vi "Read Controller Info.vi"(7 "Unit ID (A)":string="A", 8 "error in":errorcluster, 10 "Software Version":u8, 11 "VISA Session In":refnum<visa-resource-name>="Alicat") -> (0 "error out":errorcluster, 1 "Disabled Items\n(used with\"DisabledItems[]\" in the\nController Select property node)":i32[](array[numeric]), 2 "Controller Info out":T1={"Controller Full Scale"=nan, "Controller Select"=0, "Control Range"=enum."Normal"} {"Controller Select" items=["No controller"=0, "Volumetric Flow"=36, "Mass Flow"=37, "Absolute Pressure"=34, "Gauge Pressure"=38, "Differential Pressure"=39]}, 3 "VISA Session Out":refnum<visa-resource-name>)   [LabVIEW 2019]
doc: "Reads multiple registers to determine the Alicat controller settings required to run the \"Write Setpoint\" VI. Outputs the currently selected control variable, its full scale, and whether the full scale is inverted, normal, or bi-directional."
uses:
  <vilib>/Instr/_visa.llb/VISA Flush IO Buffer Mask.ctl
panel:
  # "SW Version defaults to 0. \nIf un-wired, it will call a \nsub-VI to check."
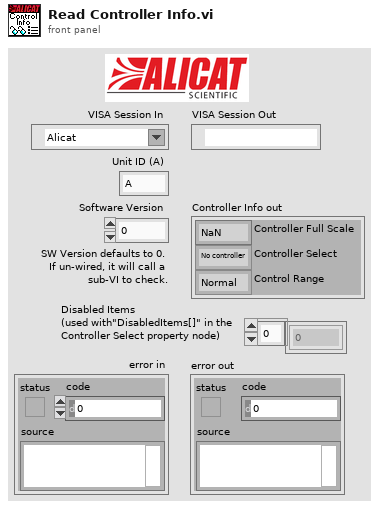
[diagram p1: front panel]
types:
  T1 = cluster{"Controller Full Scale":dbl, "Controller Select":u16, "Control Range":enum16{"Normal", "Inverted", "Bidirectional", "Unknown"}}
  T2 = cluster{"Controller Select":u16, "SetPoint Source":enum8{"Serial", "Local", "Analog", "Unknown"}, "AutoTare":enum16{"Disabled", "Enabled"}}
  T3 = cluster{"Absolute Pressure":dbl, "Gauge/Diff. Pressure":dbl, "Volumetric Flow":dbl, "Mass Flow":dbl}
  T4 = cluster{"Serial/Local Setpoint":enum8{"Don't Save", "Save"}, "FP Buttons":enum8{"Unlocked", "Locked"}, "Valve Hard Zero":enum16{"On zero setpoint", "Startup only"}, "Initial Screen":enum16{"Main", "Totalizer"}, "Gas Select":enum8{"Don't Save", "Save"}, "Tare Delay":dbl, "Control Range":enum16{"Normal", "Inverted", "Bidirectional", "Unknown"}}
  T5 = typedef "VISA Flush IO Buffer Mask.ctl" = u16
  T6 = enum16{"Normal", "Inverted", "Bidirectional", "Unknown"}
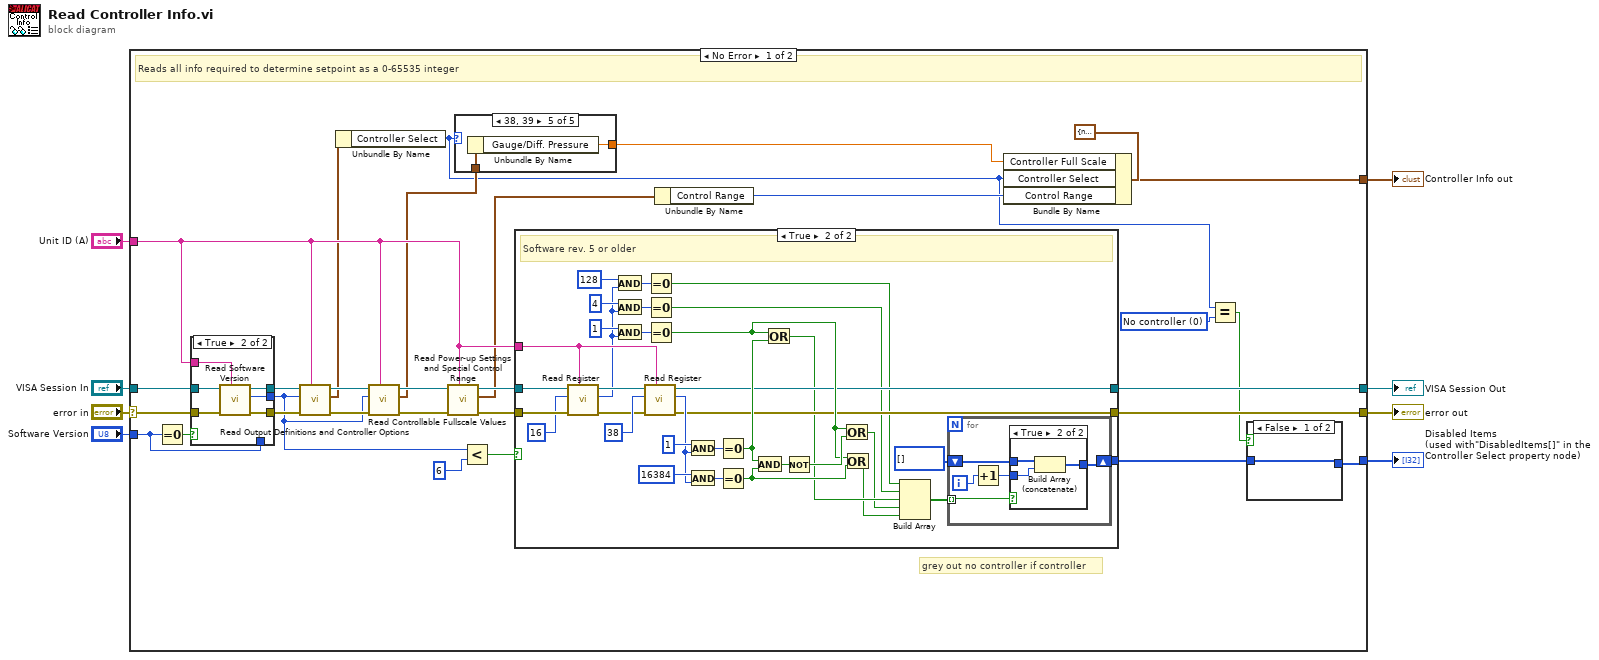
[diagram p0: block diagram]
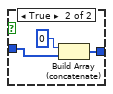
[diagram p2: hidden frame]
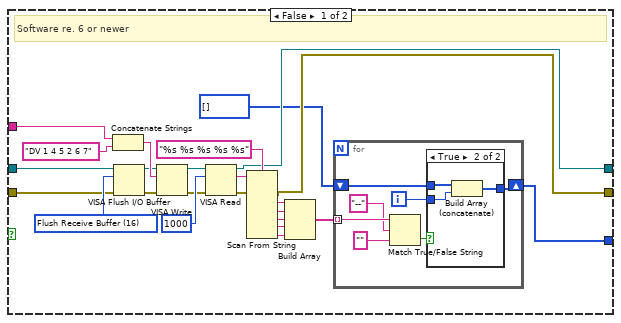
[diagram p3: hidden frame]
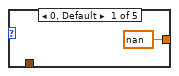
[diagram p6: hidden frame]
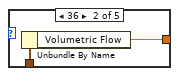
[diagram p7: hidden frame]
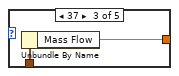
[diagram p8: hidden frame]
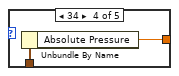
[diagram p9: hidden frame]
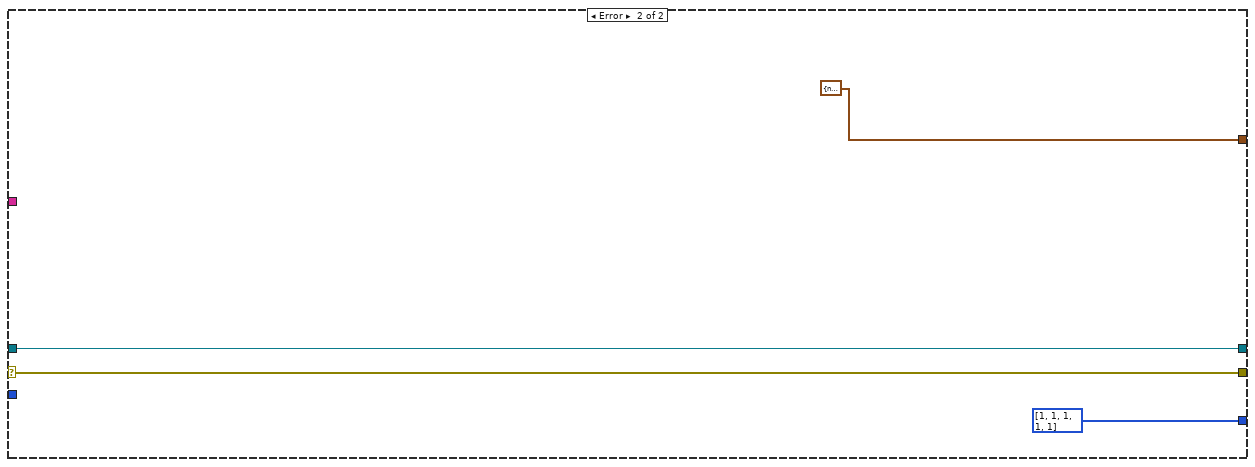
[diagram p11: hidden frame]
diagram:
  n1 = case shown="No Error" "error in" {
    selector: "error in" -> [w35 w141]
    tunnel: "VISA Session In" -> [w36 w142]
    tunnel: "Unit ID (A)" -> [w38 _]
    tunnel: [w18 w142] -> w6
    tunnel: [w19 w141] -> w5
    tunnel: [w14 T1 {"Controller Full Scale"=nan, "Controller Select"=37, "Control Range"=enum."Normal"} ("Controller Info out")] -> w1
    tunnel: "Software Version" -> [w33 _]
    tunnel: [w9 i32[] [1, 1, 1, 1, 1]] -> w2
    frame No Error {
      w13 = u16 0 items=["No controller"=0, "Volumetric Flow"=36, "Mass Flow"=37, "Absolute Pressure"=34, "Gauge Pressure"=38, "Differential Pressure"=39] ("Controller Select")
      # "grey out no controller if controller"
      # "Reads all info required to determine setpoint as a 0-65535 integer"
      n2 = Equal To 0?(x=w33) -> (x = 0?=w34:bool)
      n3 = case shown="True" w34 {
        tunnel: w35 -> [w131 w138]
        tunnel: w36 -> [w130 w137]
        tunnel: w38 -> [_ w136]
        tunnel: [w131 w135] -> w32
        tunnel: [w130 w134] -> w31
        tunnel: [w132 w133] -> w23
        tunnel: w33 -> [w132 _]
        frame False {
        }
        frame True {
          n4 = call "Read Software Version.vi"("Unit ID (A)"=w136, "error in"=w138, "VISA Session In"=w137) -> ("error out"=w135:errorcluster, "Software Version"=w133:u8, "VISA Session Out"=w134:refnum<visa-resource-name>)  [unwired: 6 in]
        }
      }
      n5 = call "Read Output Definitions and Controller Options.vi"("Unit ID (A)"=w38, "error in"=w32, "Software Version"=w23, "VISA Session In"=w31) -> ("error out"=w29:errorcluster, "Read/Write Options"=w16:T2, "VISA Session Out"=w30:refnum<visa-resource-name>)  [unwired: 4 in, 1 out]
      n6 = Unbundle By Name(w16) -> ("Controller Select"=w12:u16)
      n7 = call "Read Controllable Fullscale Values.vi"("Unit ID (A)"=w38, "error in"=w29, "Software Version"=w23, "VISA Session In"=w30) -> ("error out"=w27:errorcluster, "Fullscale"=w26:T3, "VISA Session Out"=w28:refnum<visa-resource-name>)  [unwired: 5 in]
      n8 = call "Read Power-up Settings and Special Control Range.vi"("Unit ID (A)"=w38, "error in"=w27, "VISA Session In"=w28) -> ("error out"=w20:errorcluster, "Power-up settings & special control range"=w17:T4, "VISA Session Out"=w21:refnum<visa-resource-name>)  [unwired: 6 in]
      n9 = case shown="38, 39" w12 {
        tunnel: w26 -> [_ w123 w125 w127 w129]
        tunnel: [nan ("Absolute Pressure") w122 w124 w126 w128] -> w25
        frame 0, Default {
        }
        frame 36 {
          n10 = Unbundle By Name(w123) -> ("Volumetric Flow"=w122:dbl)
        }
        frame 37 {
          n11 = Unbundle By Name(w125) -> ("Mass Flow"=w124:dbl)
        }
        frame 34 {
          n12 = Unbundle By Name(w127) -> ("Absolute Pressure"=w126:dbl)
        }
        frame 38, 39 {
          n13 = Unbundle By Name(w129) -> ("Gauge/Diff. Pressure"=w128:dbl)
        }
      }
      n14 = Less?(x=w23, y=u8 6) -> (x < y?=w22:bool)
      n15 = case shown="True" w22 {
        tunnel: w21 -> [w52 w110]
        tunnel: w20 -> [w51 w111]
        tunnel: [w50 w87] -> w19
        tunnel: [w49 w86] -> w18
        tunnel: w38 -> [w48 w105]
        tunnel: [w43 w80] -> w10
        frame False {
          w61 = T5 16 items=["Flush Receive Buffer"=16, "Write Transmit Buffer to Device"=32, "Flush Receive Buffer (No I/O)"=64, "Flush Transmit Buffer"=128] ("Mask")
          # "Software re. 6 or newer"
          n16 = Concatenate Strings(w48, "DV 1 4 5 2 6 7" ("string")) -> (w65:string)
          n17 = VISA Flush I/O Buffer(VISA resource name=w52, mask (16)=w61, error in (no error)=w51) -> (VISA resource name out=w62:refnum<visa-resource-name>, error out=w63:errorcluster)
          n18 = VISA Write(VISA resource name=w62, write buffer=w65, error in (no error)=w63) -> (VISA resource name out=w59:refnum<visa-resource-name>, error out=w58:errorcluster)  [unwired: 1 out]
          n19 = VISA Read(VISA resource name=w59, byte count=u32 1000, error in (no error)=w58) -> (VISA resource name out=w49:refnum<visa-resource-name>, read buffer=w53:string, error out=w66:errorcluster)  [unwired: 1 out]
          n20 = Scan From String(format string="%s %s %s %s %s", input string=w53, error in=w66) -> (error out=w50:errorcluster, output 1=w56:string, output 2=w55:string, output 3=w45:string, output 4=w46:string, output 5=w47:string)  [unwired: 6 in, 2 out]
          n21 = Build Array(w56, w55, w45, w46, w47) -> (w54:string[])
          n22 = for {
            tunnel: w54 -> [w73] mode=indexing
            shift-right: [w67] -> w43
            shift-left: i32[] [] -> [w69]
            i -> [w68]
            n23 = Match True/False String(2:"" ("false string"), 3:"--", 4:w73) -> (0:w70:bool)  [unwired: 1 out]
            n24 = case shown="True" w70 {
              tunnel: w69 -> [w74 w77]
              tunnel: w68 -> [_ w76]
              tunnel: [w74 w75] -> w67
              frame False {
              }
              frame True {
                n25 = Build Array (concatenate)(w77, w76) -> (w75:i32[])
              }
            }
          }
        }
        frame True {
          # "Software rev. 5 or older"
          n26 = call "Read Register.vi"("Unit ID (A)"=w105, "error in"=w111, "Register address"=u16 16, "VISA Session In"=w110) -> ("error out"=w106:errorcluster, "Register Value (I32)"=w101:i32, "VISA Session Out"=w107:refnum<visa-resource-name>)  [unwired: 5 in]
          n27 = And(x=128, y=w101) -> (x .and. y?=w97:i32)
          n28 = And(x=4, y=w101) -> (x .and. y?=w96:i32)
          n29 = And(x=1, y=w101) -> (x .and. y?=w95:i32)
          n30 = call "Read Register.vi"("Unit ID (A)"=w105, "error in"=w106, "Register address"=u16 38, "VISA Session In"=w107) -> ("error out"=w87:errorcluster, "Register Value (I32)"=w98:i32, "VISA Session Out"=w86:refnum<visa-resource-name>)  [unwired: 5 in]
          n31 = Equal To 0?(x=w97) -> (x = 0?=w85:bool)
          n32 = Equal To 0?(x=w96) -> (x = 0?=w84:bool)
          n33 = Equal To 0?(x=w95) -> (x = 0?=w89:bool)
          n34 = And(x=1, y=w98) -> (x .and. y?=w94:i32)
          n35 = And(x=16384, y=w98) -> (x .and. y?=w93:i32)
          n36 = Equal To 0?(x=w94) -> (x = 0?=w92:bool)
          n37 = Equal To 0?(x=w93) -> (x = 0?=w88:bool)
          n38 = And(x=w92, y=w88) -> (x .and. y?=w91:bool)
          n39 = Or(x=w89, y=w92) -> (x .or. y?=w83:bool)
          n40 = Not(x=w91) -> (.not. x?=w90:bool)
          n41 = Or(x=w89, y=w90) -> (x .or. y?=w82:bool)
          n42 = Or(x=w89, y=w88) -> (x .or. y?=w81:bool)
          n43 = Build Array(w85, w84, w83, w82, w81) -> (w78:bool[])
          n44 = for {
            shift-right: [w115] -> w80
            shift-left: i32[] [] -> [w116]
            tunnel: w78 -> [w114] mode=indexing
            i -> [w113]
            n45 = Increment(x=w113) -> (x+1=w112:i32)
            n46 = case shown="True" w114 {
              tunnel: w116 -> [w117 w120]
              tunnel: w112 -> [_ w119]
              tunnel: [w117 w118] -> w115
              frame False {
              }
              frame True {
                n47 = Build Array (concatenate)(w120, w119) -> (w118:i32[])
              }
            }
          }
        }
      }
      n48 = Unbundle By Name(w17) -> ("Control Range"=w37:T6)
      n49 = Bundle By Name(cluster=T1 {"Controller Full Scale"=nan, "Controller Select"=0, "Control Range"=enum."Normal"} ("Controller Info out"), "Controller Full Scale"=w25, "Controller Select"=w12, "Control Range"=w37) -> (w14:T1)
      n50 = Equal?(x=w12, y=w13) -> (x = y?=w11:bool)
      n51 = case shown="False" w11 {
        tunnel: w10 -> [w39 w42]
        tunnel: [w39 w40] -> w9
        frame False {
        }
        frame True {
          n52 = Build Array (concatenate)(0, w42) -> (w40:i32[])
        }
      }
    }
    frame Error {
    }
  }
  "error out" <- w5
  "VISA Session Out" <- w6
  "Controller Info out" <- w1
  "Disabled Items\n(used with\"DisabledItems[]\" in the\nController Select property node)" <- w2
